vi "Convert RPM.vi"(8 "Velocity (m/s)":dbl, 11 "Velocity (RPM)":dbl) -> (0 "Velocity (RPM)":dbl, 3 "Velocity (m/s)":dbl)   [LabVIEW 2020]
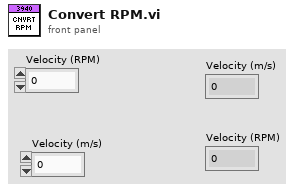
[diagram p1: front panel]
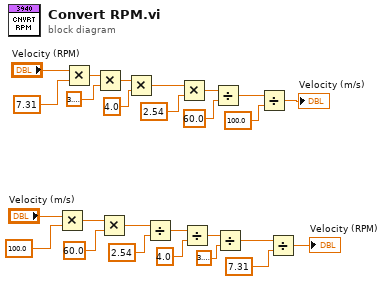
[diagram p0: block diagram]
diagram:
  n1 = Multiply(x="Velocity (m/s)", y=100.0) -> (x*y=w11:dbl)
  n2 = Multiply(x="Velocity (RPM)", y=7.31) -> (x*y=w24:dbl)
  n3 = Multiply(x=w24, y=3.141592653589793) -> (x*y=w22:dbl)
  n4 = Multiply(x=w11, y=60.0) -> (x*y=w9:dbl)
  n5 = Multiply(x=w22, y=4.0) -> (x*y=w20:dbl)
  n6 = Divide(x=w9, y=2.54) -> (x/y=w7:dbl)
  n7 = Multiply(x=w20, y=2.54) -> (x*y=w18:dbl)
  n8 = Divide(x=w7, y=4.0) -> (x/y=w5:dbl)
  n9 = Divide(x=w18, y=60.0) -> (x/y=w16:dbl)
  n10 = Divide(x=w5, y=3.141592653589793) -> (x/y=w3:dbl)
  n11 = Divide(x=w16, y=100.0) -> (x/y=→"Velocity (m/s)":dbl)
  n12 = Divide(x=w3, y=7.31) -> (x/y=→"Velocity (RPM)":dbl)
